vi "Create Registry.vi"(8 "error in":errorcluster) -> (0 "error out":errorcluster, 3 "Registry":refnum<data-value>)   [LabVIEW 2019, in "Identifier.lvclass"]
uses:
  Identifier.lvclass
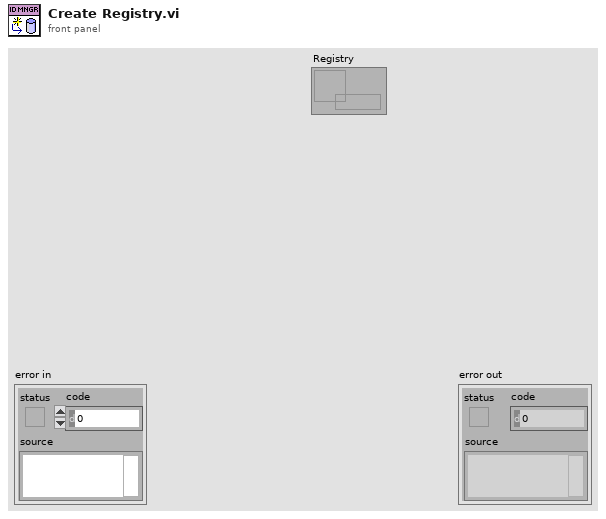
[diagram p1: front panel]
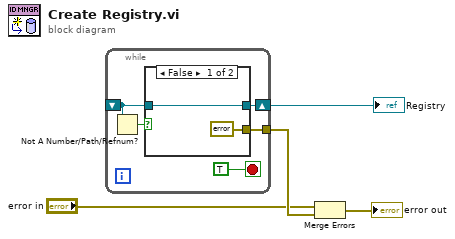
[diagram p0: block diagram]
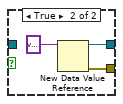
[diagram p2: hidden frame]
diagram:
  n1 = while {
    shift-right: [w8] -> w1
    shift-left: _ -> [w6]
    tunnel: [w5] -> w4
    stop <- TRUE stop-if-true
    n2 = Not A Number/Path/Refnum?(number/path/refnum=w6) -> (NaN/Path/Refnum?=w9:bool)
    n3 = case shown="False" w9 {
      tunnel: w6 -> [w11 _]
      tunnel: [w11 w13] -> w8
      tunnel: [errorcluster {"status"=FALSE, "code"=0, "source"=""} ("error out") w12] -> w5
      frame False {
      }
      frame True {
        n4 = New Data Value Reference(data value=variant) -> (data value reference=w13:refnum<data-value>, error out=w12:errorcluster)  [unwired: 1 in]
      }
    }
  }
  "Registry" <- w1
  n5 = Merge Errors("error in", w4) -> (→"error out":errorcluster)
